vi "PID Joint Position Control.vi"() -> ()   [LabVIEW 2018]
uses:
  <vilib>/Platform/TimedLoop/XDataNode/timing_clust.ctl
  <vilib>/Platform/TimedLoop/XDataNode/nitl_modes.ctl
  <vilib>/Platform/TimedLoop/XDataNode/wakeup.ctl
  <vilib>/Platform/TimedLoop/XDataNode/XDataNode.xnode
  <vilib>/Platform/TimedLoop/XDataNode/XDNodeRunTimeDep.lvlib
panel:
  out "Error":errorcluster
  in  "Stop Button":bool
  out "Calibrated":bool
  out "Voltage Command (V)":dbl(graph)
  out "Motor Angles (rad)":T1(graph)
  out "Theta 0 percentage error":dbl
  in  "Integral (ki)":dbl=0.9999999999999999 min=0.0 max=100.0 step=0.1
  in  "Derivative (kd)":dbl=1.0 min=0.0 max=5.0 step=0.1
  in  "Proportional (kp)":dbl=5.0 min=0.0 max=100.0 step=0.1
  # "Engineering Trainer Boards"
  # "Mechatronic Systems\nPID Joint Position Control"
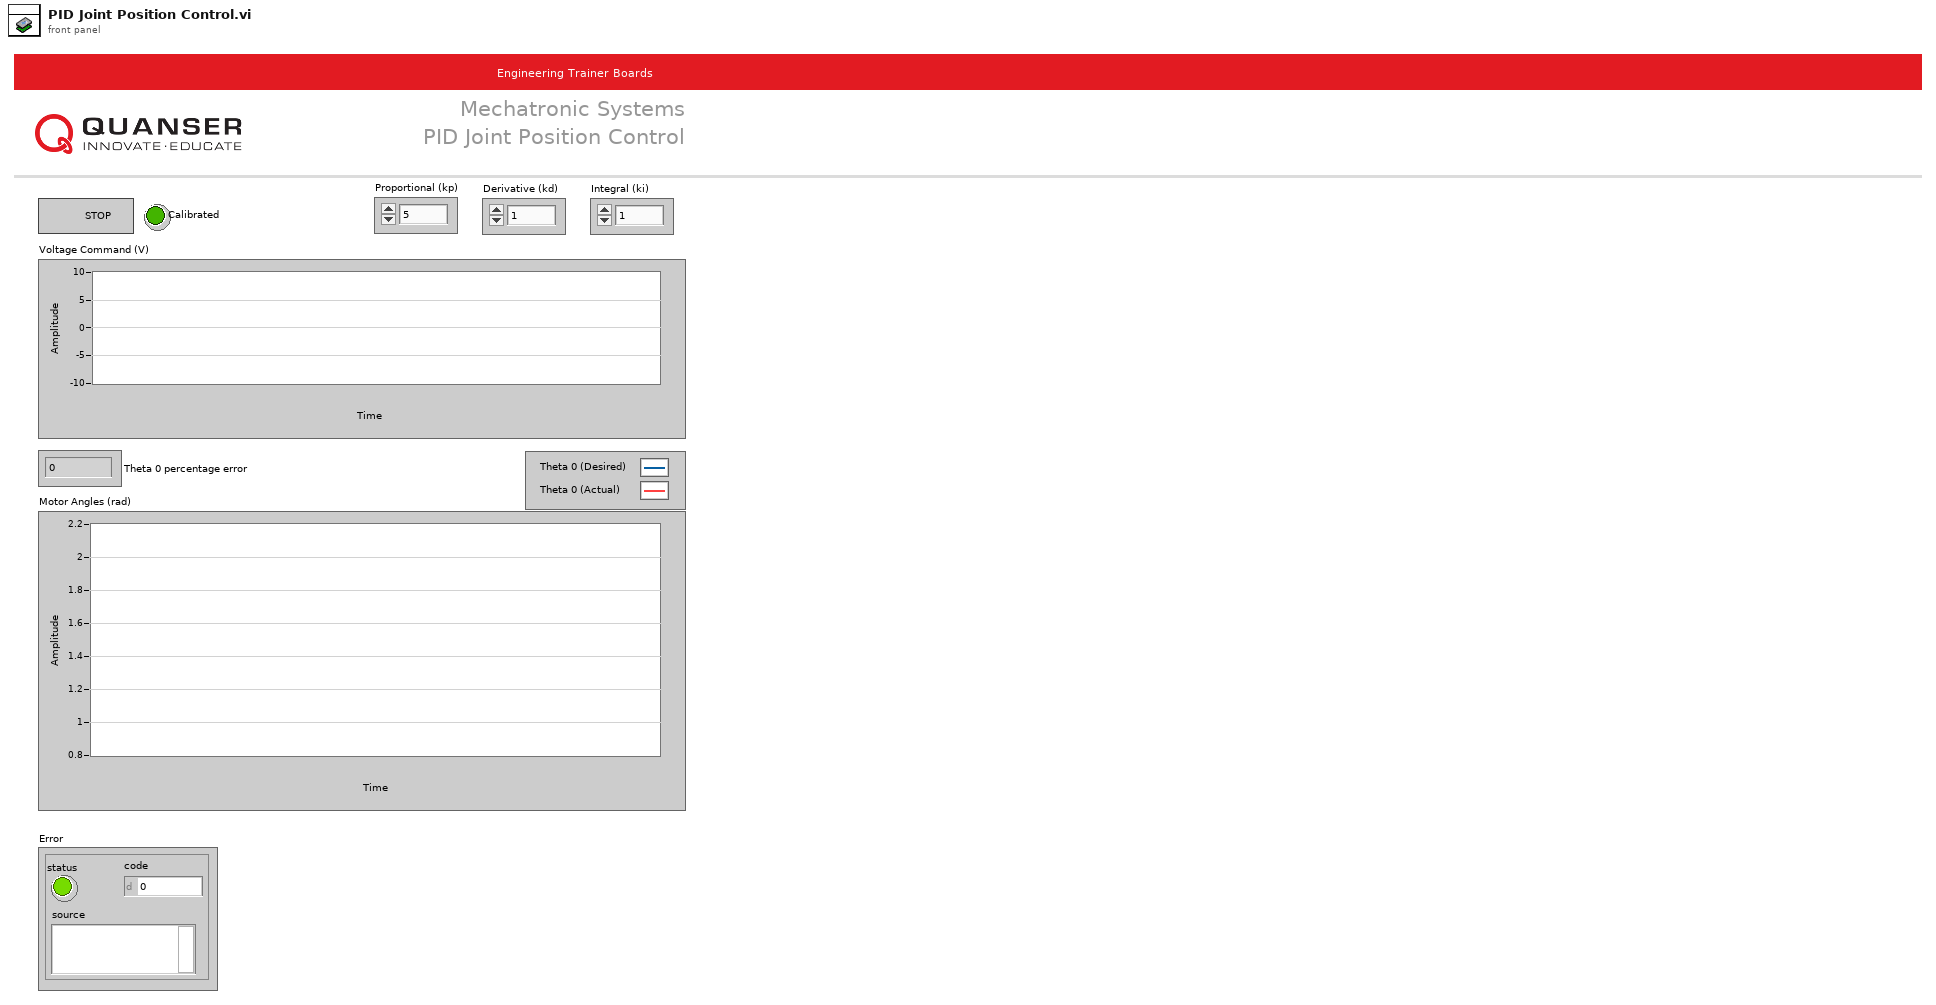
[diagram p1: front panel]
types:
  T1 = cluster{"f":dbl, "Numeric Control":dbl, "element":dbl, "element 2":dbl, "element 3":dbl, "element 4":dbl}
  T2 = typedef "XDNodeRunTimeDep.lvlib/timing_clust.ctl" = cluster{"Expected End [f-1]":u64, "Actual End [f-1]":u64, "Finished Late? [f-1]":bool, "Expected End [i-1]":u64, "Actual End [i-1]":u64, "Finished Late? [i-1]":bool, "Expected Start [i]":u64, "Actual Start [i]":u64, "Expected Start [f]":u64, "Actual Start [f]":u64, "Source Name":string, "Structure Name":string, "Period":i64, "Deadline":i64, "Offset":i64, "Start":i64, "Priority":i32, "Timeout":i32, "Mode":T3, "Wakeup Reason":T4, "Error":errorcluster, "Source Type":string, "Secondary Source Type":string, "Global End Time":u64, "Global Start Time":u64, "Frame Duration":u64, "Iteration Duration":u64, "Assigned CPU":i32, "I/O Scan Engine Mode":u32}
  T3 = typedef "XDNodeRunTimeDep.lvlib/nitl_modes.ctl" = enum32{"No Change", "Process missed periods, maintain original phase", "Discard missed periods, maintain original phase", "Process missed periods, ignore original phase", "Discard missed periods, ignore original phase"}
  T4 = typedef "XDNodeRunTimeDep.lvlib/wakeup.ctl" = enum32{"Normal", "Aborted", "Asynchronous wakeup", "Timing source error", "Timed loop error", "Timeout"}
  T5 = typedef "QNET MS IO Cluster.ctl" = cluster{"Error":errorcluster, "Encoder Calibration Values":i32[], "Update Calibration":bool, "JPEG Resolutions":u16, "Raw Resolutions":u16, "Image Mode":enum16{"RAW RGB", "RAW Gray Scale", "JPEG"}, "FPGA Ref":refnum<k20>}
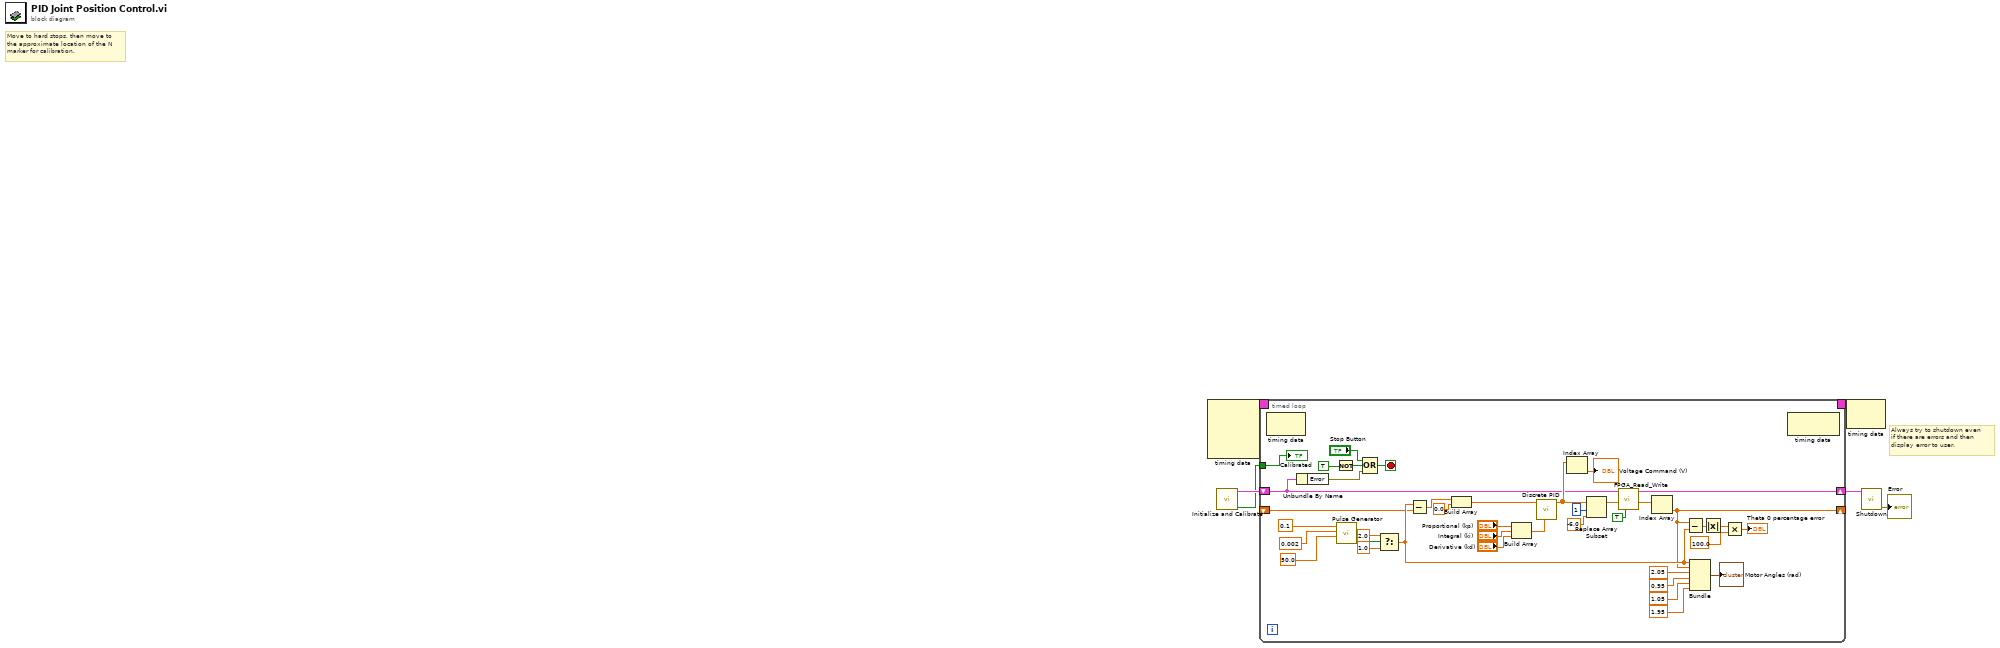
[diagram p0: block diagram]
diagram:
  # "Always try to shutdown even \nif there are errors and then \ndisplay error to user."
  # "Move to hard stops, then move to\nthe approximate location of the N\nmarker for calibration."
  n1 = node-c288() -> (w6:T2)  [unwired: 4 in]
  n2 = call "Initialize and Calibrate.vi"() -> ("Calibrated"=w3:bool, "IO Cluster"=w4:T5)  [unwired: 10 in]
  n3 = timed-loop {
    timing: w6 -> [_]
    timing-out: [_] -> w5
    shift-right: [w8] -> _
    shift-left: _ -> [w24]
    tunnel: w3 -> [w16]
    shift-right: [w15] -> w2
    shift-left: w4 -> [w18]
    stop <- w17 stop-if-true
    n4 = node-c288() -> ()  [unwired: 1 in, 1 out]
    n5 = Unbundle By Name(w18) -> ("Error"=w14:errorcluster)
    n6 = Not(x=TRUE) -> (.not. x?=w13:bool)
    n7 = call "Pulse Generator.vi"("Duty Cycle"=50.0, "Step size"=0.002, "Frequency"=0.1 ("Desired pulse frequency (Hz)")) -> ("Pulse Wave"=w43:bool)  [unwired: 5 in, 3 out]
    n8 = Compound Arithmetic op=OR("Stop Button", w13, w14) -> (w17:bool)
    n9 = Select(t=2.0, s=w43, f=1.0) -> (s? t:f=w25:dbl)
    n10 = Subtract(x=w25, y=w24) -> (x-y=w10:dbl)
    n11 = Build Array ("Build Array 2")(w10, 0.0 ("Error 1")) -> (w39:dbl[])
    n12 = Build Array ("Build Array 3")("Proportional (kp)", "Integral (ki)", "Derivative (kd)") -> (w40:dbl[])
    n13 = call "Discrete PID.vi"("Gains Motor 0"=w40, "Error Array"=w39) -> ("Voltage"=w19:dbl[])  [unwired: 9 in]
    n14 = Index Array ("Index Array 2")(array=w19) -> (element=→"Voltage Command (V)":dbl)  [unwired: 1 in]
    n15 = Replace Array Subset(array=w19, new element=-6.0 ("new element/subarray"), index=1) -> (w22:dbl[])
    n16 = call "FPGA_Read_Write.vi"("Motors enabled?"=TRUE ("Motors Enabled"), "Commands"=w22, "IO Cluster In"=w18) -> ("Joint Coordinates (rad)"=w34:dbl[], "IO Cluster Out"=w15:T5)  [unwired: 5 in, 2 out]
    n17 = Index Array(array=w34) -> (element=w8:dbl)  [unwired: 1 in]
    n18 = Subtract ("Subtract 2")(x=w8, y=w25) -> (x-y=w30:dbl)
    n19 = Bundle("f"=w25, "Numeric Control"=w8, "element"=2.05, "element 2"=0.95, "element 3"=1.05, "element 4"=1.95) -> (→"Motor Angles (rad)":T1)  [unwired: 1 in]
    n20 = Absolute Value(x=w30) -> (abs(x)=w31:dbl)
    n21 = Multiply(x=w31, y=100.0) -> (x*y=→"Theta 0 percentage error":dbl)
    n22 = node-c288() -> ()  [unwired: 1 in, 1 out]
    "Calibrated" <- w16
  }
  n23 = node-c288(w5) -> ()  [unwired: 1 out]
  n24 = call "Shutdown.vi"("IO Cluster In"=w2) -> ("Error"=→"Error":errorcluster)  [unwired: 10 in]
